vi "InstrumentObjectArray_write_and_unlock.vi"(8 "error in (no error)":errorcluster, 11 "InstrumentObjects":refnum<class "instrument.lvclass">[](array[class])) -> (0 "error out":errorcluster)   [LabVIEW 2017]
doc: "the VI writes and unlocks the InstrumentObjectsArray using a Queue"
uses:
  Classes/Instrument/instrument.lvclass
  global variables.vi
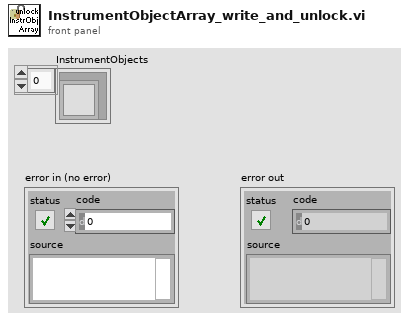
[diagram p1: front panel]
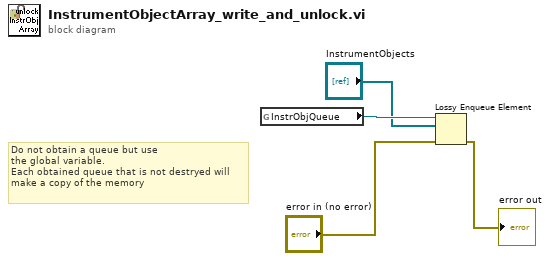
[diagram p0: block diagram]
diagram:
  # "Do not obtain a queue but use\nthe global variable.\nEach obtained queue that is not destryed will\nmake a copy of the memory"
  n1 = global read "global variables.vi" "InstrObjQueue"() -> (w3:refnum<queue>)
  n2 = Lossy Enqueue Element(queue=w3, element="InstrumentObjects", error in (no error)="error in (no error)") -> (error out=→"error out":errorcluster)  [unwired: 3 out]
